vi "Get All Test Events.vi"(8 "error in (no error)":errorcluster, 11 "Test Event Storage in":refnum<class "Test Event Storage.lvclass">) -> (0 "error out":errorcluster, 1 "Test Events":T1[](array[typedef]), 2 "Parent Keys":string[](array[string]), 3 "Test Event Storage out":refnum<class "Test Event Storage.lvclass">)   [LabVIEW 2013, in "Caraya.lvlib" / "Test Event Storage.lvclass"]
uses:
  Test Event Storage.lvclass
  Test Result/Assert Event Data.ctl
  Test Event Storage.lvclass/Test Event Storage.ctl
  Test Result/Test Result.lvclass
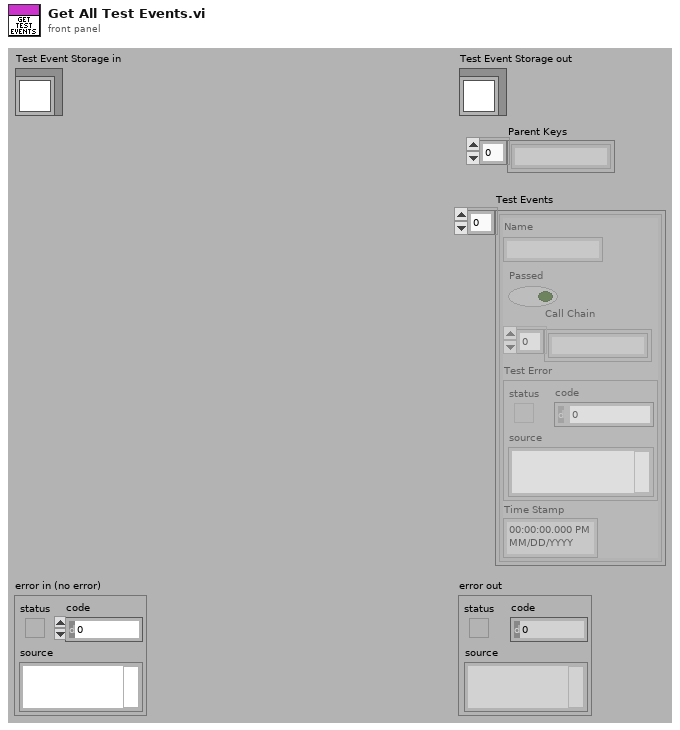
[diagram p1: front panel]
types:
  T1 = typedef "Caraya.lvlib/Test Result.lvclass/Assert Event Data.ctl" = cluster{"Name":string, "Passed":bool, "Call Chain":string[], "Test Error":errorcluster, "Time Stamp":timestamp}
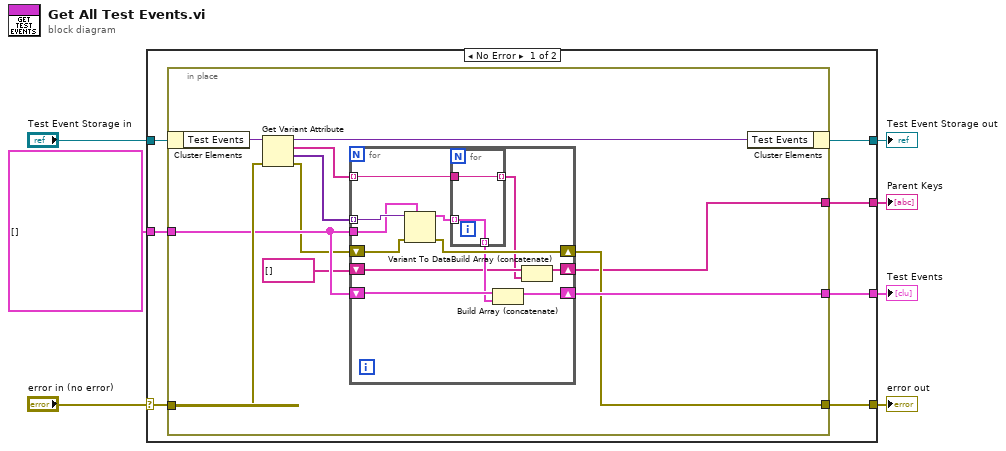
[diagram p0: block diagram]
diagram:
  n1 = case shown="No Error" "error in (no error)" {
    selector: "error in (no error)" -> [w11 w41]
    tunnel: [w14 w41] -> w6
    tunnel: [w13 w40] -> w4
    tunnel: "Test Event Storage in" -> [w12 w40]
    tunnel: T1[] [] -> [w10 _]
    tunnel: [w9 _] -> w2
    tunnel: [w8 _] -> w1
    frame No Error {
      n2 = in-place {
        in-place-border: w11 -> [w24]
        in-place-border: [w18] -> w14
        in-place-border: w10 -> [w21]
        in-place-border: [w20] -> w9
        in-place-border: [w15] -> w8
        n3 = in-place-cluster #1(w12) -> ("Test Events"=w25:variant)
        n4 = Get Variant Attribute(Variant=w25, error in=w24) -> (duplicate Variant=w23:variant, names=w17:string[], values=w22:variant[], error out=w19:errorcluster)  [unwired: 2 in]
        n5 = for {
          tunnel: w22 -> [w37] mode=indexing
          tunnel: w21 -> [w36]
          shift-right: [w34] -> w18
          shift-left: w19 -> [w35]
          shift-right: [w33] -> w20
          shift-left: w21 -> [w32]
          tunnel: w17 -> [w31] mode=indexing
          shift-right: [w27] -> w15
          shift-left: string[] [] -> [w28]
          n6 = Variant To Data(error in=w35, type=w36, Variant=w37) -> (data=w29:T1[], error out=w34:errorcluster)
          n7 = for {
            tunnel: w31 -> [w38]
            tunnel: [w39] -> w30 mode=indexing
            tunnel: w29 -> [w39] mode=indexing
            tunnel: [w38] -> w26 mode=indexing
          }
          n8 = Build Array (concatenate)(w32, w30) -> (w33:T1[])
          n9 = Build Array (concatenate)(w28, w26) -> (w27:string[])
        }
        n10 = in-place-cluster #1("Test Events"=w23) -> (w13:refnum<class "Test Event Storage.lvclass">)
      }
    }
    frame Error {
    }
  }
  "error out" <- w6
  "Test Event Storage out" <- w4
  "Test Events" <- w2
  "Parent Keys" <- w1
